vi "Model.vi"() -> ()   [LabVIEW 2026]
uses:
  <vilib>/DAQmx/read.llb/DAQmx Read (Analog 1D Wfm NChan NSamp).vi
  <vilib>/DAQmx/create/channels.llb/DAQmx Create Channel (AI-Voltage-Basic).vi
  <vilib>/DAQmx/configure/timing.llb/DAQmx Timing (Sample Clock).vi
  <vilib>/DAQmx/configure/task.llb/DAQmx Configure Logging (TDMS).vi
  <vilib>/DAQmx/miscellaneous.llb/DAQmx Fill In Error Info.vi
  <resource>/objmgr/daqmx.rc
panel:
  in  "physical channels":tag
  in  "y":bool
  out "error out":errorcluster
  out "Waveform Graph 2":waveform(dbl)(graph)
  out "Waveform Graph":waveform(dbl)(graph)
  in  "operation":i32(ring)=15846 items=["Open"=10437, "Open or Create"=15846, "Create or Replace"=15847, "Create"=15848]
  in  "group name":string
  in  "logging mode":i32(ring)=15842 items=["Off"=10231, "Log"=15844, "Log and Read"=15842]
  in  "file path":path
  in  "rate":dbl=1000.0 format="%0.2f"
  in  "samples per channel":i32=1000
  in  "sample mode":i32(ring)=10178 items=["Finite Samples"=10178, "Continuous Samples"=10123, "Hardware Timed Single Point"=12522]
  in  "input terminal configuration":i32(ring)=-1 items=["Default"=-1, "RSE"=10083, "NRSE"=10078, "Differential"=10106, "Pseudodifferential"=12529]
  in  "minimum value":dbl=-5.0 format="%0.2f"
  in  "maximum value":dbl=5.0 format="%0.2f"
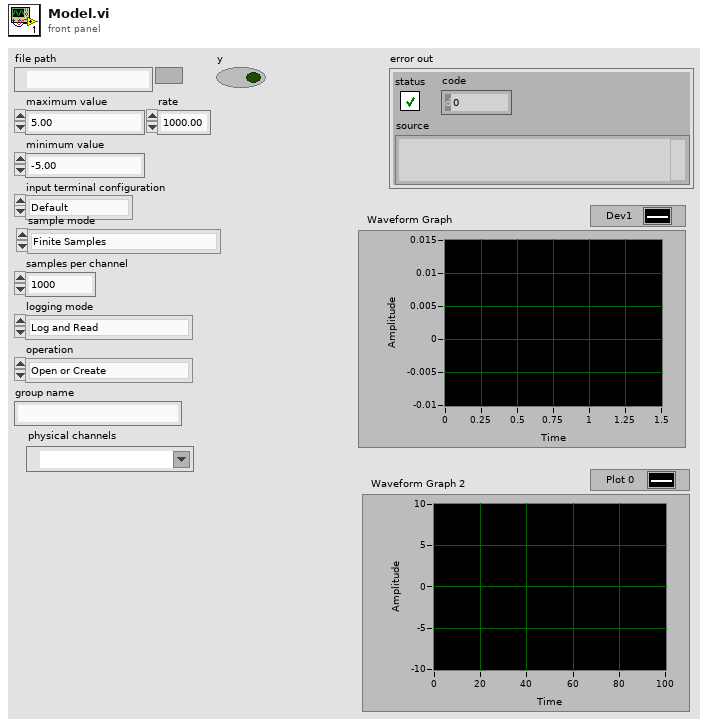
[diagram p1: front panel]
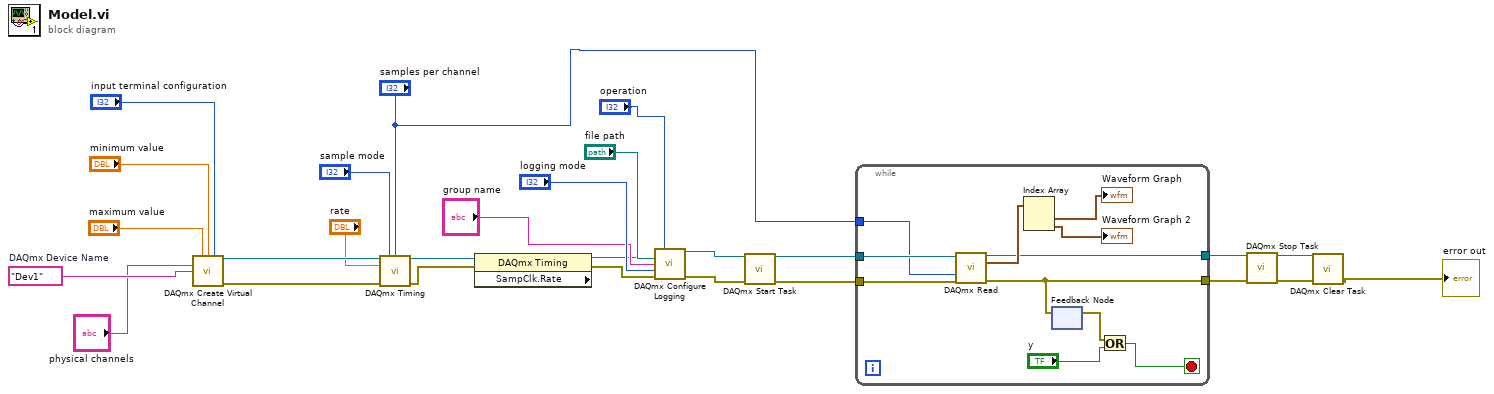
[diagram p0: block diagram]
diagram:
  w2 = tag "Dev1"  # DAQmx Device Name
  n1 = call-poly <vilib>:"DAQmx Create Virtual Channel.vi"("maximum value"="maximum value", "minimum value"="minimum value", "input terminal configuration"="input terminal configuration", "physical channels"="physical channels", "name to assign"=w2) -> ("task out"=w24:refnum<k21>, "error out"=w23:errorcluster)  [unwired: 9 in]
  n2 = call-poly <vilib>:"DAQmx Timing.vi"("task/channels in"=w24, "sample mode"="sample mode", "samples per channel"="samples per channel", "rate"="rate", "error in"=w23) -> ("task out"=w18:refnum<k21>, "error out"=w17:errorcluster)  [unwired: 9 in]
  n3 = property class="DAQmx Timing" props=["SampClk.Rate"](reference=w18, error in=w17) -> (reference out=w12:refnum<k21>, error out=w16:errorcluster)  [unwired: 1 out]
  n4 = call-poly <vilib>:"DAQmx Configure Logging.vi"("task/channels in"=w12, "operation"="operation", "file path"="file path", "group name"="group name", "logging mode"="logging mode", "error in"=w16) -> ("task out"=w19:refnum<k21>, "error out"=w20:errorcluster)  [unwired: 8 in]
  n5 = call <vilib>:"DAQmx Start Task.vi"("task/channels in"=w19, "error in"=w20) -> ("task out"=w10:refnum<k21>, "error out"=w9:errorcluster)  [unwired: 12 in]
  n6 = while {
    tunnel: w10 -> [w38]
    tunnel: w9 -> [w37]
    tunnel: "samples per channel" -> [w36]
    tunnel: [w30] -> w4
    tunnel: [w34] -> w3
    stop <- w33 stop-if-true
    n7 = call-poly <vilib>:"DAQmx Read.vi"("task/channels in"=w38, "timeout"=w36, "error in"=w37) -> ("task out"=w34:refnum<k21>, "data"=w35:waveform(dbl)[], "error out"=w30:errorcluster)  [unwired: 10 in]
    n8 = Index Array(array=w35) -> (element #1=→"Waveform Graph":waveform(dbl), element #2=→"Waveform Graph 2":waveform(dbl))  [unwired: 2 in]
    n9 = feedback-in #1(w30) -> ()
    n10 = feedback #1() -> (w31:errorcluster)  [unwired: 1 in]
    n11 = Or(x=w31, y="y") -> (x .or. y?=w33:bool)
  }
  n12 = call <vilib>:"DAQmx Stop Task.vi"("task/channels in"=w3, "error in"=w4) -> ("task out"=w7:refnum<k21>, "error out"=w6:errorcluster)  [unwired: 12 in]
  n13 = call <vilib>:"DAQmx Clear Task.vi"("task in"=w7, "error in"=w6) -> ("error out"=→"error out":errorcluster)  [unwired: 13 in]
